vi "CreateLabVIEWItemObject.vi"(8 "error in (no error)":errorcluster, 10 "delimited name":string, 11 "SubVI path":path) -> (0 "error out":errorcluster, 3 "ILabVIEWItem":refnum<class "ILabVIEWItem.lvclass">)   [LabVIEW 2020, in "LabVIEWObjectFactory.lvlib"]
uses:
  LabVIEWObjectFactory.lvlib
  obj/Addons/LabVIEWObjectInterfaces.lvlibp/LabVIEWObjectInterfaces/ILabVIEWItem/ILabVIEWItem.lvclass
  obj/Addons/LabVIEWFiles.lvlibp/CLabVIEWItemOtherFile/CLabVIEWItemOtherFile.lvclass
  C:/DependencyInspector/obj/Addons/LabVIEWItem.lvlibp/LabVIEWItem/CLabVIEWItem/CLabVIEWItem.lvclass
  obj/Addons/LabVIEWFiles.lvlibp/CLabVIEWItemVI/CLabVIEWItemVI.lvclass
  obj/Addons/LabVIEWFiles.lvlibp/CLabVIEWItemCtl/CLabVIEWItemCtl.lvclass
  obj/Addons/LabVIEWContainers.lvlibp/LabVIEWContainers/CLabVIEWItemLibrary/CLabVIEWItemLibrary.lvclass
  obj/Addons/LabVIEWContainers.lvlibp/LabVIEWContainers/CLabVIEWItemClass/CLabVIEWItemClass.lvclass
  obj/Addons/LabVIEWContainers.lvlibp/LabVIEWContainers/CLabVIEWItemXControl/CLabVIEWItemXControl.lvclass
  obj/Addons/LabVIEWFiles.lvlibp/CLabVIEWItemVIM/CLabVIEWItemVIM.lvclass
  obj/Addons/LabVIEWFiles.lvlibp/CLabVIEWItemBadFile/CLabVIEWItemBadFile.lvclass
  obj/Addons/LabVIEWItem.lvlibp/LabVIEWItem/CLabVIEWItem/CLabVIEWItem.lvclass
  C:/DependencyInspector/obj/Addons/LabVIEWObjectInterfaces.lvlibp/LabVIEWObjectInterfaces/ILabVIEWItem/ILabVIEWItem.lvclass
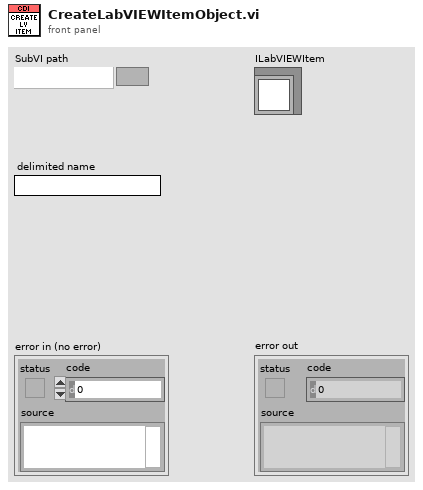
[diagram p1: front panel]
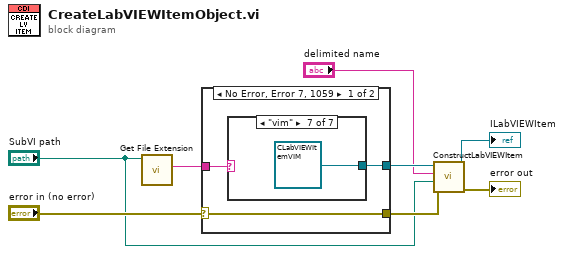
[diagram p0: block diagram]
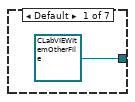
[diagram p2: hidden frame]
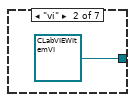
[diagram p3: hidden frame]
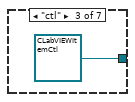
[diagram p4: hidden frame]
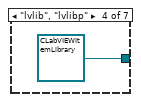
[diagram p5: hidden frame]
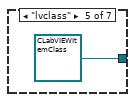
[diagram p6: hidden frame]
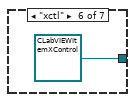
[diagram p7: hidden frame]
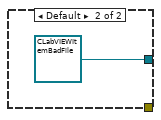
[diagram p8: hidden frame]
diagram:
  n1 = call <vilib>:"Get File Extension.vi"("file"="SubVI path") -> ("lowercase file extension"=w8:string)  [unwired: 6 in, 4 out]
  n2 = case shown="No Error, Error 7, 1059" "error in (no error)" {
    selector: "error in (no error)" -> [w9 _]
    tunnel: w8 -> [w11 _]
    tunnel: [w10 refnum<class "CLabVIEWItemBadFile.lvclass"> refnum ("DGML_Generator_Helper.lvlib:CLabVIEWItemBadFile.lvclass")] -> w7
    tunnel: [w9 _] -> w2
    frame No Error {
      n3 = case shown="\"vim\"" w11 {
        tunnel: [refnum<class "CLabVIEWItemOtherFile.lvclass"> refnum ("DGML_Generator_Helper.lvlib:CLabVIEWItemOtherFile.lvclass") refnum<class "CLabVIEWItemVI.lvclass"> refnum ("DGML_Generator_Helper.lvlib:CLabVIEWItemVI.lvclass") refnum<class "CLabVIEWItemCtl.lvclass"> refnum ("DGML_Generator_Helper.lvlib:CLabVIEWItemCtl.lvclass") refnum<class "CLabVIEWItemLibrary.lvclass"> refnum ("DGML_Generator_Helper.lvlib:CLabVIEWItemLibrary.lvclass") refnum<class "CLabVIEWItemClass.lvclass"> refnum ("DGML_Generator_Helper.lvlib:CLabVIEWItemClass.lvclass") refnum<class "CLabVIEWItemXControl.lvclass"> refnum ("DGML_Generator_Helper.lvlib:CLabVIEWItemXControl.lvclass") refnum<class "CLabVIEWItemVIM.lvclass"> refnum ("DGML_Generator_Helper.lvlib:CLabVIEWItemVIM.lvclass")] -> w10
        frame Default {
        }
        frame "vi" {
        }
        frame "ctl" {
        }
        frame "lvlib", "lvlibp" {
        }
        frame "lvclass" {
        }
        frame "xctl" {
        }
        frame "vim" {
        }
      }
    }
    frame Default {
    }
  }
  n4 = call-dynamic "ConstructLabVIEWItem.vi"("error in (no error)"=w2, "Path"="SubVI path", "Qualified name"="delimited name", "CLabVIEWItem in"=w7) -> ("error out"=→"error out":errorcluster, "CLabVIEWItem out"=→"ILabVIEWItem":refnum<class "CLabVIEWItem.lvclass">)  [unwired: 6 in]
